vi "LFU Convert End Of Line__ogtk.vi"(2 "convert to LV":bool, 3 "input":string) -> (1 "output":string)   [LabVIEW 2018]
doc: "Low level utility function to convert EOLs."
panel:
  # "[OpenG VI Tags] ***Do Not Remove***"
  # "LFU Convert End Of Line.vi\n\nPlease visit http://www.OpenG.org to learn about the\nOpen Source LabVIEW software movement.\n\nNOTICE -- YOU MUST LEAVE THIS NOTICE IN PLACE.  PER THE TERMS OF THE LICENSE BELOW, YOU MAY SUBLICENSE THIS SOFTWARE \nIN ANY WAY THAT DOES NOT CONFLICT WITH THIS LICENSE.\n\n### BSD License (http://www.opensource.org/licenses/bsd-license.php) Begin ###\n\nCopyright (c) 2003, Rolf Kalbermatter <rolf.kalbermatter@citeng.com>\n\nAll rights reserved.\n\nRedistribution and use in source and binary forms, with or without modification, are permitted provided that the following conditions are met:\n\n    * Redistributions of source code must retain the above copyright notice, this list of conditions and the following disclaimer.\n    * Redistributions in binary form must reproduce the above copyright notice, this list of conditions and the following disclaimer in the \n       documentation and/or other materials provided with the distribution.\n    * Neither the name of SciWare, James Kring, Inc., nor the names of its contributors may be used to endorse or promote products derived \n       from this software without specific prior written permission.\n\nTHIS SOFTWARE IS PROVIDED BY THE COPYRIGHT HOLDERS AND CONTRIBUTORS \"AS IS\" AND ANY EXPRESS OR IMPLIED WARRANTIES, \nINCLUDING, BUT NOT LIMITED TO, THE IMPLIED WARRANTIES OF MERCHANTABILITY AND FITNESS FOR A PARTICULAR PURPOSE ARE \nDISCLAIMED. IN NO EVENT SHALL THE COPYRIGHT OWNER OR CONTRIBUTORS BE LIABLE FOR ANY DIRECT, INDIRECT, INCIDENTAL,\n SPECIAL, EXEMPLARY, OR CONSEQUENTIAL DAMAGES (INCLUDING, BUT NOT LIMITED TO, PROCUREMENT OF SUBSTITUTE GOODS OR \nSERVICES; LOSS OF USE, DATA, OR PROFITS; OR BUSINESS INTERRUPTION) HOWEVER CAUSED AND ON ANY THEORY OF LIABILITY, \nWHETHER IN CONTRACT, STRICT LIABILITY, OR TORT (INCLUDING NEGLIGENCE OR OTHERWISE) ARISING IN ANY WAY OUT OF THE USE \nOF THIS SOFTWARE, EVEN IF ADVISED OF THE POSSIBILITY OF SUCH DAMAGE.\n\n### BSD License End ###"
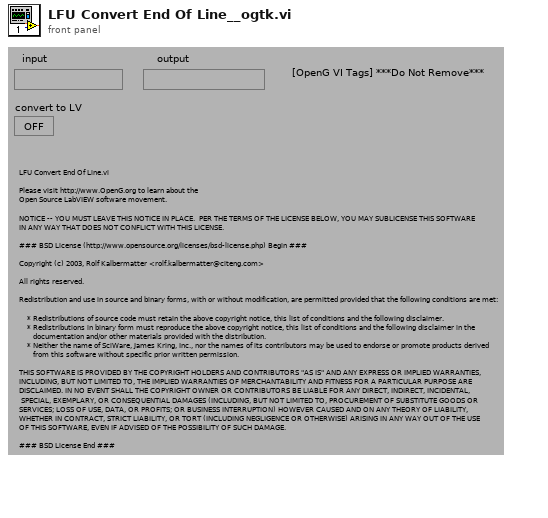
[diagram p1: front panel]
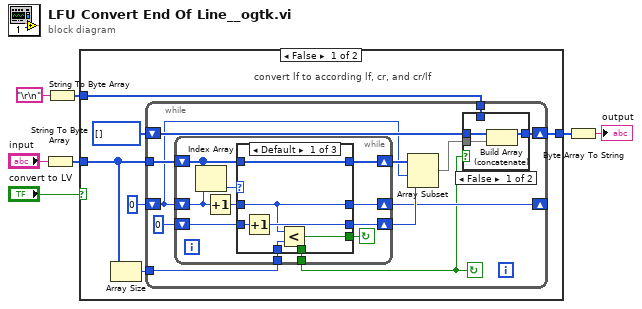
[diagram p0: block diagram]
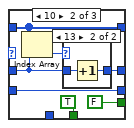
[diagram p2: hidden frame]
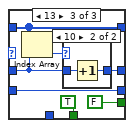
[diagram p4: hidden frame]
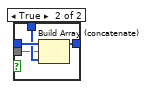
[diagram p6: hidden frame]
diagram:
  n1 = String To Byte Array(string="input") -> (unsigned byte array=w1:u8[])
  n2 = String To Byte Array(string="\r\n") -> (unsigned byte array=w2:u8[])
  n3 = case shown="False" "convert to LV" {
    tunnel: w1 -> [w9 w70]
    tunnel: [w11 w70] -> w3
    tunnel: w2 -> [w10 _]
    frame False {
      # "convert lf to according lf, cr, and cr/lf"
      n4 = Array Size(array=w9) -> (size(s)=w8:i32)
      n5 = while {
        tunnel: w8 -> [w20]
        tunnel: w10 -> [w23]
        shift-left: u8[] [] ("input") -> [w24]
        shift-right: [w25] -> w11
        tunnel: w9 -> [w22]
        shift-left: 0 -> [w18]
        shift-right: [w15] -> _
        stop <- w14 continue-if-true
        n6 = while {
          tunnel: [w26] -> w14
          tunnel: w20 -> [w27]
          shift-left: 0 -> [w30]
          shift-right: [w29] -> w17
          shift-left: w22 -> [w33]
          shift-right: [w32] -> w19
          shift-left: w18 -> [w36]
          shift-right: [w31] -> w15
          stop <- w28 continue-if-true
          n7 = Index Array(array=w33, index=w36) -> (element=w35:u8)
          n8 = Increment(x=w36) -> (x+1=w34:i32)
          n9 = case shown="Default" w35 {
            tunnel: w34 -> [w39 w48 w58]
            tunnel: w33 -> [w42 w49 w59]
            tunnel: [w42 w49 w59] -> w32
            tunnel: [w39 w47 w57] -> w31
            tunnel: w30 -> [w41 w44 w54]
            tunnel: [w40 w44 w54] -> w29
            tunnel: [w37 FALSE FALSE] -> w28
            tunnel: w27 -> [w38 _ _]
            tunnel: [w37 TRUE TRUE] -> w26
            frame Default {
              n10 = Increment(x=w41) -> (x+1=w40:i32)
              n11 = Less?(x=w39, y=w38) -> (x < y?=w37:bool)
            }
            frame 10 {
              n12 = Index Array(array=w49, index=w48) -> (element=w46:u8)
              n13 = case shown="13" w46 {
                tunnel: w48 -> [w50 w52]
                tunnel: [w50 w51] -> w47
                frame Default {
                }
                frame 13 {
                  n14 = Increment(x=w52) -> (x+1=w51:i32)
                }
              }
            }
            frame 13 {
              n15 = Index Array(array=w59, index=w58) -> (element=w56:u8)
              n16 = case shown="10" w56 {
                tunnel: w58 -> [w60 w62]
                tunnel: [w60 w61] -> w57
                frame Default {
                }
                frame 10 {
                  n17 = Increment(x=w62) -> (x+1=w61:i32)
                }
              }
            }
          }
        }
        n18 = Array Subset(array=w19, index=w18, length=w17) -> (w16:u8[])
        n19 = case shown="False" w14 {
          tunnel: [w64 w69] -> w25
          tunnel: w24 -> [w65 w68]
          tunnel: w23 -> [_ w67]
          tunnel: w16 -> [w63 w66]
          frame False {
            n20 = Build Array (concatenate)(w65, w63) -> (w64:u8[])
          }
          frame True {
            n21 = Build Array (concatenate)(w68, w66, w67) -> (w69:u8[])
          }
        }
      }
    }
    frame True {
      # "convert lf, cr, and cr/lf to lf"
    }
  }
  n22 = Byte Array To String(unsigned byte array=w3) -> (string=→"output":string)
